vi "final temp pressure rec.vi"() -> ()   [LabVIEW 2025]
panel:
  out "Pressure(psia)":dbl
  out "Pressure Graph":dynamicdata(graph)
  out "Pressure Chart":dynamicdata(graph)
  out "Temperature Graph":dynamicdata(graph)
  out "Temperature Chart":dynamicdata(graph)
  out "Temperature(deg C)":dbl
  in  "stop":bool
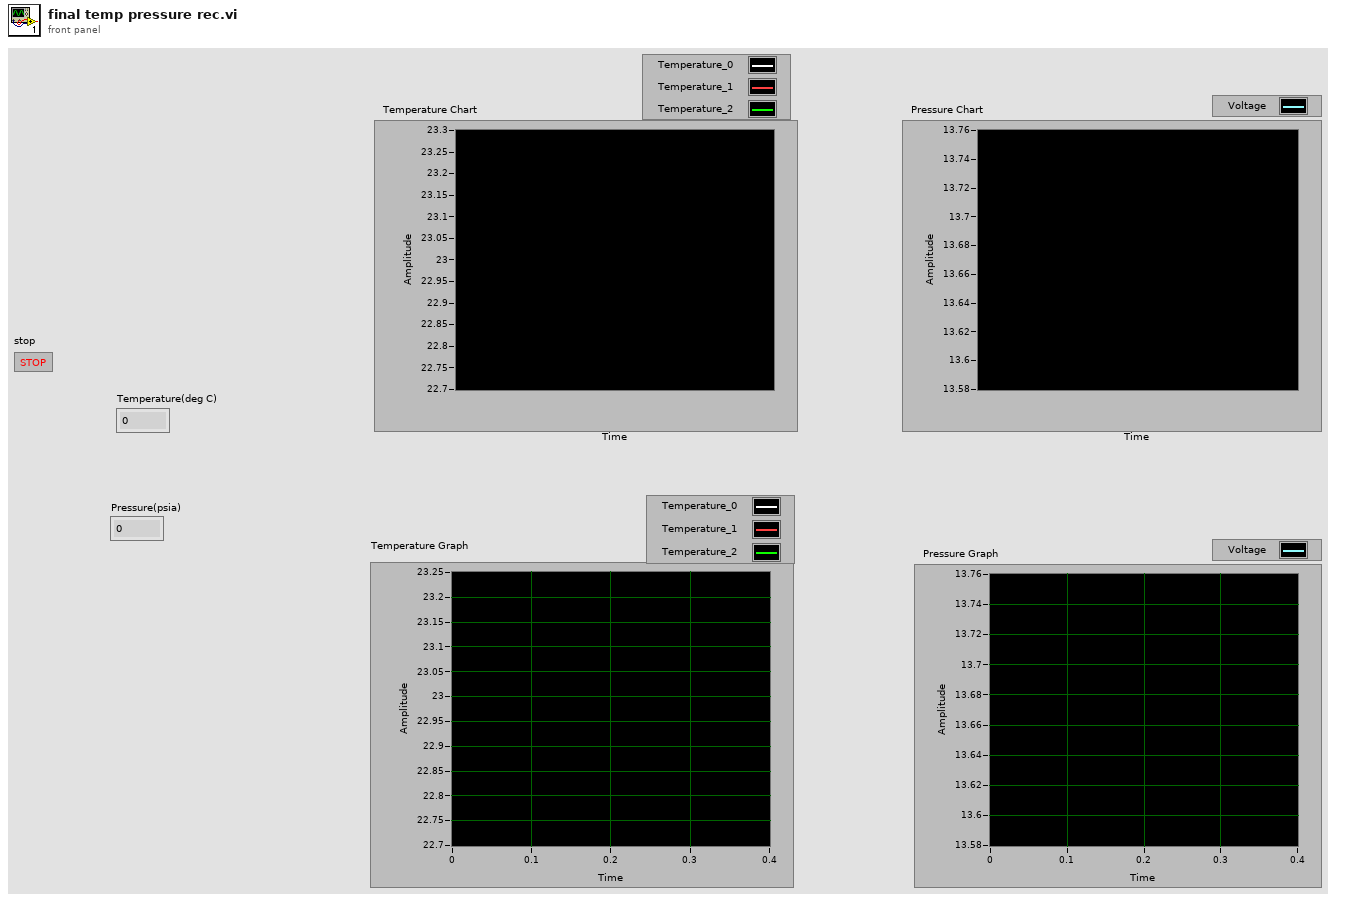
[diagram p1: front panel]
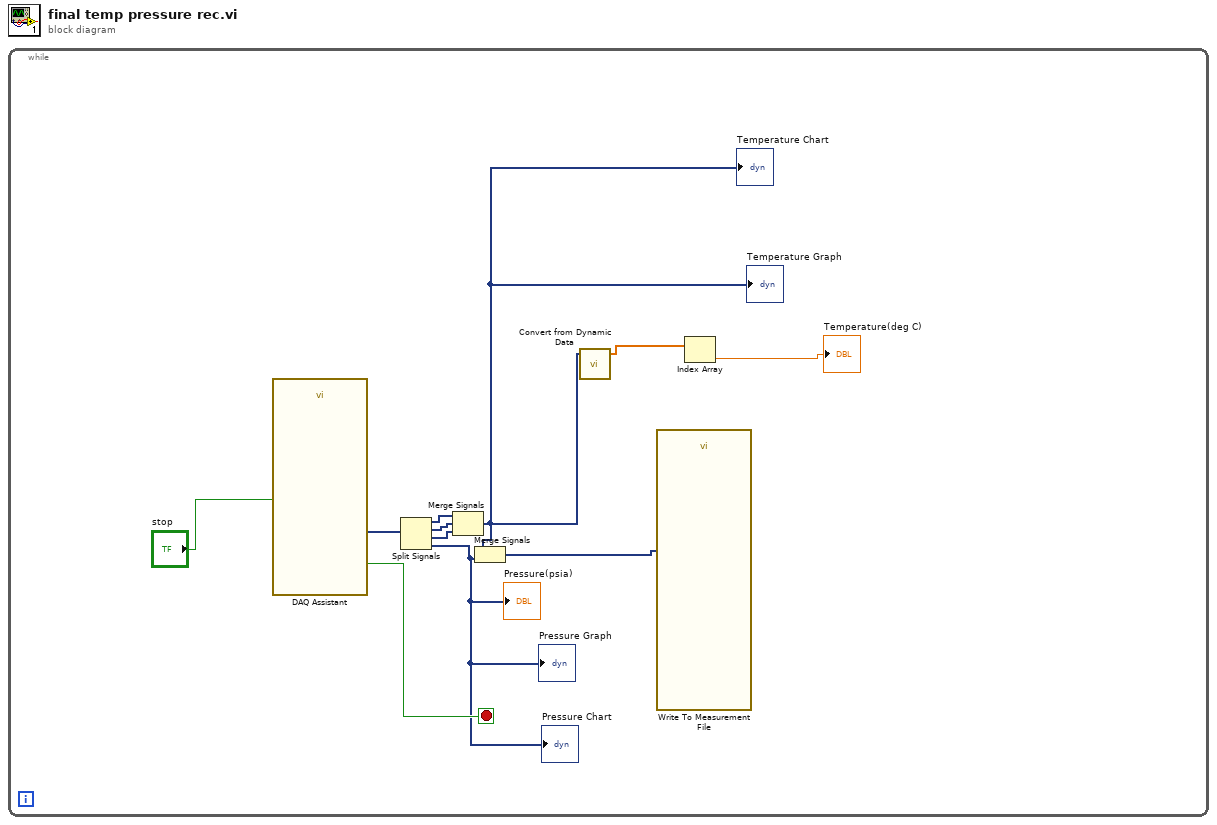
[diagram p0: block diagram]
diagram:
  n1 = while {
    stop <- w10 stop-if-true
    n2 = call "DAQ Assistant"("stop (F)"="stop") -> ("data"=w9:dynamicdata, "stopped"=w10:bool)  [unwired: 15 in, 2 out]
    n3 = Split Signals(w9) -> (w8:dynamicdata, w7:dynamicdata, w6:dynamicdata, w1:dynamicdata)  [unwired: 4 in]
    "Pressure(psia)" <- w1
    "Pressure Chart" <- w1
    "Pressure Graph" <- w1
    n4 = Merge Signals(w8, w7, w6) -> (w5:dynamicdata)
    "Temperature Chart" <- w5
    "Temperature Graph" <- w5
    n5 = Merge Signals(w5, w1) -> (w2:dynamicdata)
    n6 = call "Convert from Dynamic Data"("Dynamic Data Type"=w5) -> ("Array"=w4:dbl[])  [unwired: 3 in]
    n7 = call "Write To Measurement File"("Signals"=w2) -> ()  [unwired: 16 in, 3 out]
    n8 = Index Array(array=w4) -> (element=→"Temperature(deg C)":dbl)  [unwired: 1 in]
  }
